vi "Saklar lampu kelap kelip.vi"() -> ()   [LabVIEW 2015]
panel:
  in  "Switch After Relased":bool
  out "Boolean 3":bool
  in  "?":bool
  out "Boolean 2":bool
  in  "Switch When Pressed":bool
  out "Boolean":bool
  # "Switch When Relased"
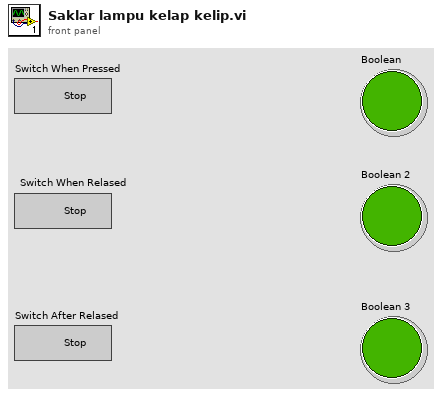
[diagram p1: front panel]
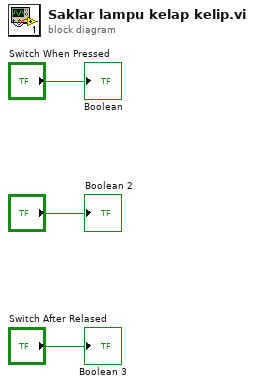
[diagram p0: block diagram]
diagram:
  "Boolean" <- "Switch When Pressed"
  "Boolean 2" <- "?"
  "Boolean 3" <- "Switch After Relased"
